vi "_049.vi"() -> ()   [LabVIEW 2024]
panel:
  out "reversed":string
  in  "string":string
  out "String 4":string
  in  "String 3":string
  out "String 2":string
  in  "String":string
  # "Reverse a String :"
  # "(using reverse 1-D Array &\n without using Reverse String)"
  # "Reverse a String :"
  # "(without using reverse 1-D Array & Reverse String)"
  # "Reverse a String :"
  # "(using Reverse String)"
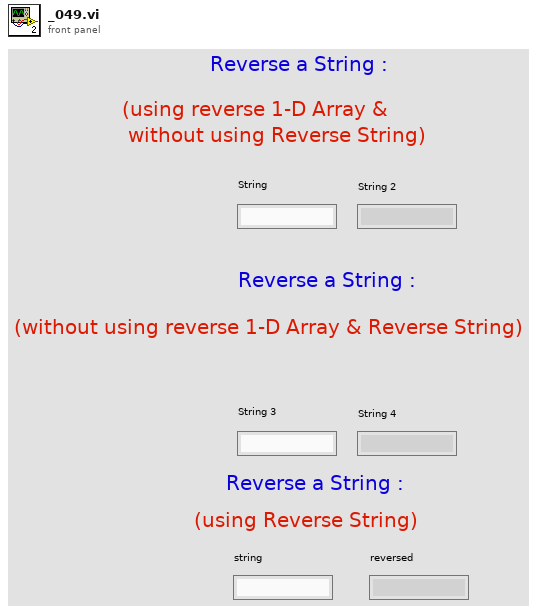
[diagram p1: front panel]
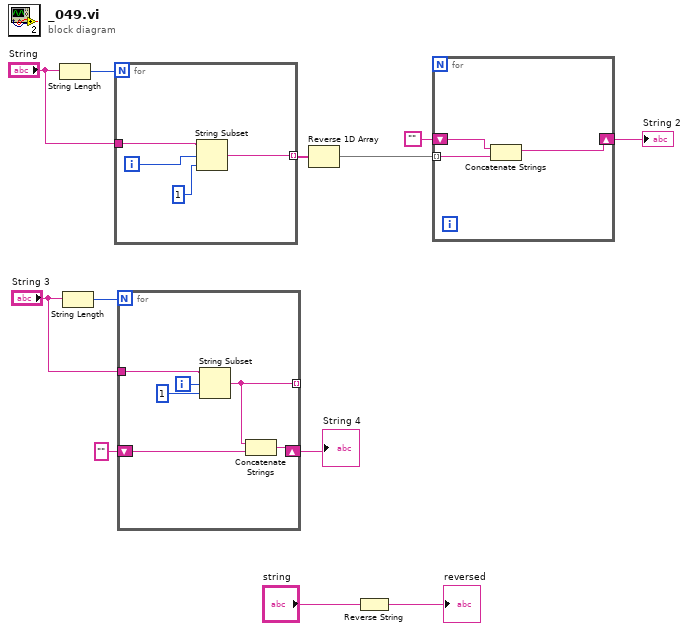
[diagram p0: block diagram]
diagram:
  n1 = String Length(string="String") -> (length=w12:i32)
  n2 = String Length(string="String 3") -> (length=w6:i32)
  n3 = for {
    N: w12 -> [_]
    tunnel: "String" -> [w16]
    tunnel: [w13] -> w10 mode=indexing
    i -> [w14]
    n4 = String Subset(string=w16, offset (0)=w14, length (rest)=1 ("length (rest)")) -> (substring=w13:string)
  }
  n5 = for {
    N: w6 -> [_]
    tunnel: "String 3" -> [w22]
    tunnel: [w19] -> _ mode=indexing
    shift-right: [w17] -> w3
    shift-left: "" -> [w18]
    i -> [w20]
    n6 = String Subset(string=w22, offset (0)=w20, length (rest)=1 ("length (rest)")) -> (substring=w19:string)
    n7 = Concatenate Strings(w19, w18) -> (w17:string)
  }
  "String 4" <- w3
  n8 = Reverse 1D Array(array=w10) -> (reversed array=w7:string[])
  n9 = Reverse String(1:"string") -> (0:→"reversed":string)
  n10 = for {
    tunnel: w7 -> [w24] mode=indexing
    shift-right: [w25] -> w8
    shift-left: "" -> [w23]
    n11 = Concatenate Strings "Concatenate Strings"(w23, w24) -> (w25:string)
  }
  "String 2" <- w8
